vi "xiLIB - PRM_Info.vi"() -> ()   [LabVIEW 2018]
uses:
  Typedefs/xiLIB - PRM_Type.ctl
  Typedefs/xiLIB - PRM_Function.ctl
  xiCam/PRM/PRM/PRM_v2.ctl
panel:
  in  "PRM[]_v2":T1[](array[typedef])=[enum."DEVICE_NAME", enum."DEVICE_TYPE", enum."DEVICE_SN", enum."EXPOSURE", enum."EXPOSURE_MAX", enum."EXPOSURE_MIN", enum."GAIN", enum."GAIN_MAX", enum."GAIN_MIN", enum."DOWNSAMPLING_TYPE", enum."DOWNSAMPLING", enum."DOWNSAMPLING_MAX", enum."DOWNSAMPLING_MIN", enum."IMAGE_DATA_FORMAT", enum."IMAGE_IS_COLOR", enum."COLOR_FILTER_ARRAY", enum."FRAMERATE", enum."FRAMERATE_MAX", enum."FRAMERATE_MIN", enum."BUFFER_POLICY", enum."OFFSET_X", enum."OFFSET_X_MAX", enum."OFFSET_X_MIN", enum."OFFSET_Y", enum."OFFSET_Y_MAX", enum."OFFSET_Y_MIN", enum."WIDTH", enum."WIDTH_MAX", enum."WIDTH_MIN", enum."HEIGHT", enum."HEIGHT_MAX", enum."HEIGHT_MIN", enum."LUT_EN", enum."LUT_INDEX", enum."LUT_INDEX_MAX", enum."LUT_INDEX_MIN", enum."LUT_VALUE", enum."LUT_VALUE_MAX", enum."LUT_VALUE_MIN", enum."TRG_SOURCE", enum."TRG_SOFTWARE", enum."GPI_SELECTOR", enum."GPI_SELECTOR_MAX", enum."GPI_SELECTOR_MIN", enum."GPI_LEVEL", enum."GPI_MODE", enum."GPO_SELECTOR", enum."GPO_SELECTOR_MAX", enum."GPO_SELECTOR_MIN", enum."GPO_MODE", enum."LED_SELECTOR", enum."LED_SELECTOR_MAX", enum."LED_SELECTOR_MIN", enum."LED_MODE", enum."ACQ_BUFFER_SIZE", enum."BUFFERS_QUEUE_SIZE", enum."WB_KR", enum."WB_KG", enum."WB_KB", enum."MANUAL_WB", enum."AUTO_WB", enum."GAMMAY", enum."GAMMAC", enum."SHARPNESS", enum."CC_MATRIX_00", enum."CC_MATRIX_01", enum."CC_MATRIX_02", enum."CC_MATRIX_03", enum."CC_MATRIX_10", enum."CC_MATRIX_11", enum."CC_MATRIX_12", enum."CC_MATRIX_13", enum."CC_MATRIX_20", enum."CC_MATRIX_21", enum."CC_MATRIX_22", enum."CC_MATRIX_23", enum."CC_MATRIX_30", enum."CC_MATRIX_31", enum."CC_MATRIX_32", enum."CC_MATRIX_33", enum."CC_MATRIX_33", enum."AEAG", enum."EXP_PRIORITY", enum."AE_MAX_LIMIT", enum."AG_MAX_LIMIT", enum."AEAG_LEVEL", enum."BPC", enum."DEBOUNCE_EN", enum."DEBOUNCE_T0", enum."DEBOUNCE_T1", enum."DEBOUNCE_POL", enum."IS_COOLED", enum."COOLING", enum."TARGET_TEMP", enum."CHIP_TEMP", enum."LED_SELECTOR_MIN", enum."HDR", enum."LIMIT_BANDWIDTH_MAX", enum."API_VERSION", enum."LUT_EN", enum."AVAILABLE_BANDWIDTH", enum."LIMIT_BANDWIDTH", enum."ACQ_BUFFER_SIZE_UNIT", enum."ACQ_TRANSPORT_BUFFER_COMMIT", enum."AEAG_ROI_HEIGHT", enum."AEAG_ROI_OFFSET_X", enum."AEAG_ROU_OFFSET_Y", enum."AEAG_ROI_WIDTH", enum."SHUTTER_TYPE", enum."GAIN_SELECTOR", enum."SENSOR_FEATURE_SELECTOR", enum."SENSOR_FEATURE_VALUE", enum."OUTPUT_DATA_BIT_DEPTH", enum."IMAGE_DATA_BIT_DEPTH", enum."SENSOR_DATA_BIT_DEPTH", enum."SENSOR_CLOCK_FREQ_HZ", enum."SENSOR_CLOCK_FREQ_INDEX", enum."OUTPUT_DATA_PACKING", enum."OUTPUT_DATA_PACKING_TYPE", enum."TRANSPORT_PIXEL_FORMAT", enum."IMAGE_PAYLOAD_SIZE", enum."SENSOR_TAPS", enum."COLUMN_FPN_CORRECTION", enum."BINNING_HORIZONTAL", enum."BINNING_SELECTOR", enum."BINNING_SELECTOR", enum."BINNING_VERTICAL", enum."DECIMATION_HORIZONTAL", enum."DECIMATION_VERTICAL", enum."DECIMATION_SELECTOR", enum."DECIMATION_VERTICAL"]
  in  "ERROR_CODE[]":i32[](array[numeric])=[0, 1, 2, 3, 4, 5, 6, 7, 8, 9, 10, 11, 12, 13, 14, 15, 16, 17, 18, 19, 20, 21, 22, 23, 24, 25, 26, 27, 28, 29, 30, 31, 32, 33, 34, 35, 36, 38, 39, 40, 41, 42, 43, 44, 45, 46, 47, 48, 49, 50, 51, 52, 53, 54, 55, 100, 101, 103, 104, 105, 106, 107, 108, 109, 110, 111]
  in  "ERROR_DESC[]":string[](array[string])=["Function call succeeded", "Invalid handle", "Register read error", "Register write error", "Freeing resiurces error", "Freeing channel error", "Freeing bandwith error", "Read block error", "Write block error", "No image", "Timeout", "Invalid arguments supplied", "Not supported", "Attach buffers error", "Overlapped result", "Memory allocation error", "DLL context is NULL", "DLL context is non zero", "DLL context exists", "Too many devices connected", "Camera context error", "Unknown hardware", "Invalid TM file", "Invalid TM tag", "Incomplete TM", "Bus reset error", "Not implemented", "Shading too bright", "Shading too dark", "Gain is too low", "Invalid bad pixel list", "Bad pixel list realloc error", "Invalid pixel list", "Invalid Flash File System", "Invalid profile", "Invalid calibration", "Invalid buffer", "Invalid data", "Timing generator is busy", "Wrong operation open/write/read/close", "Acquisition already started", "Old version of device driver installed to the system.", "To get error code please call GetLastError function.", "Data can't be processed", "Acquisition has been stopped. It should be started before GetImage.", "Acquisition has been stoped with error.", "Input ICC profile missed or corrupted", "Output ICC profile missed or corrupted", "Device not ready to operate", "Shading too contrast", "Modile already initialized", "Application doesn't enough privileges(one or more app", "Installed driver not compatible with current software", "TM file was not loaded successfully from resources", "Device has been reseted, abnormal initial state", "Unknown parameter", "Wrong parameter value", "Wrong parameter type", "Wrong parameter size", "Input buffer too small", "Parameter info not supported", "Parameter info not supported", "Data format not supported", "Read only parameter", "No devices found", "This camera does not support currently available bandwidth"]
  in  "PRM-Method[]":T2[](array[typedef])=[enum."Get", enum."Get", enum."Get", enum."Get / Set", enum."Get", enum."Get", enum."Get / Set", enum."Get", enum."Get", enum."Get / Set", enum."Get / Set", enum."Get", enum."Get", enum."Get / Set", enum."Get", enum."Get", enum."Get", enum."Get", enum."Get", enum."Get / Set", enum."Get / Set", enum."Get", enum."Get", enum."Get / Set", enum."Get", enum."Get", enum."Get / Set", enum."Get", enum."Get", enum."Get / Set", enum."Get", enum."Get", enum."Get / Set", enum."Get / Set", enum."Get", enum."Get", enum."Get / Set", enum."Get", enum."Get", enum."Get / Set", enum."Set", enum."Get / Set", enum."Get", enum."Get", enum."Get", enum."Get / Set", enum."Get / Set", enum."Get", enum."Get", enum."Get / Set", enum."Get / Set", enum."Get", enum."Get", enum."Get / Set", enum."Get / Set", enum."Get / Set", enum."Get / Set", enum."Get / Set", enum."Get / Set", enum."Set", enum."Get / Set", enum."Get / Set", enum."Get / Set", enum."Get / Set", enum."Get / Set", enum."Get / Set", enum."Get / Set", enum."Get / Set", enum."Get / Set", enum."Get / Set", enum."Get / Set", enum."Get / Set", enum."Get / Set", enum."Get / Set", enum."Get / Set", enum."Get / Set", enum."Get / Set", enum."Get / Set", enum."Get / Set", enum."Get / Set", enum."Set", enum."Get / Set", enum."Get / Set", enum."Get / Set", enum."Get / Set", enum."Get / Set", enum."Get / Set", enum."Get / Set", enum."Get / Set", enum."Get / Set", enum."Get / Set", enum."Get", enum."Get", enum."Get", enum."Get", enum."Get", enum."Get / Set", enum."Get / Set", enum."Get", enum."Get", enum."Get", enum."Get", enum."Get / Set", enum."Get / Set", enum."Get / Set", enum."Get / Set", enum."Get / Set", enum."Get / Set", enum."Get / Set", enum."Get / Set", enum."Get / Set", enum."Get / Set", enum."Get / Set", enum."Get / Set", enum."Get / Set", enum."Get / Set", enum."Get / Set", enum."Get / Set", enum."Get / Set", enum."Get / Set", enum."Get", enum."Get / Set", enum."Get / Set", enum."Get / Set", enum."Get / Set", enum."Get / Set", enum."Get / Set", enum."Get / Set", enum."Get / Set", enum."Get / Set", enum."Get / Set"]
  in  "PRM-Desc[]":string[](array[string])=["Get camera model name.", "Returns device type (1394, USB2.0, CURRERA…..).", "Returns device serial number in decimal format.", "Set/Get exposure time in microseconds.", "Get longest possible exposure to be set on camera.", "Get shortest possible exposure to be set on camera.", "Set/Get camera gain in dB.", "Get highest possible camera gain in dB.", "Get lowest possible camera gain in dB.", "BINNING: Pixels are interpoled - better image, SKIPPING: pixels are skipped - higher framerate", "Changes image resolution, where one image pixel is: '1' - sensor pixel , '2' - 2x2 , '4' - 4x4.", "Get highest value for binning or skipping.", "Get lowest value for binning or skipping", "Set/Get output image data format. Use class IMG_FORMAT to set value.", "Returns 1 for color cameras", "Returns color filter array type of RAW data.", "Get frames per second.", "Get highest possible framerate for current camera settings.", "Get lowest framerate for current camera settings", "Data move policy", "Set/Get horizontal offset from the origin to the area of interest (in pixels).", "Get maximum horizontal offset from the origin to the area of interest (in pixels).", "Get minimum horizontal offset from the origin to the area of interest (in pixels).", "Set/Get vertical offset from the origin to the area of interest (in pixels).", "Get maximum vertical offset from the origin to the area of interest (in pixels).", "Get minimal vertical offset from the origin to the area of interest (in pixels). ", "Set/Get width of the image provided by the camera (in pixels)", "Get maximal image width provided by the camera (in pixels).", "Get minimal image width provided by the camera (in pixels)", "Set/Get height of the image provided by the camera (in pixels).", "Get maximal image height provided by the camera (in pixels).", "Get minimal image height provided by the camera (in pixels). ", "Activates look up table. Currently available only for Currera-R cameras.", "Controls the index (offset) of the coefficient to access in the LUT.", "Get highest LUT index (offset) of the coefficient to access in the LUT. ", "Get lowest LUT index (offset) of the coefficient to access in the LUT.", "Set/Get value at entry LUTIndex of the LUT.", "Get highest value to be set in LUT.", "Get lowest value to be set in LUT.", "Set/Get source of trigger. Use TRG_SOURCE class to set parameter.", "Set an internal software trigger. PRM.TRG_SOURCE must be set to TRG_SOFTWARE", "Select camera GPI port.", "Get highest GPI port number on camera.", "Get lowest GPI port number on camera.", "Get current GPI level", "Set/Get GPI functionality. Select port by using GPI_SELECTOR parameter. ", "Select camera GPO port", "Get highest GPO port number on camera.", "Get lowest GPI port number on camera", "Set/Get GPO functionality. Select port by using GPO_SELECTOR parameter.", "Selects camera LED to be used. Currently supported only for Currera-R cameras.", "Get highest LED number on camera", "Get lowest LED number on camera", "Set/Get LED functionality. Select port by using LED_SELECTOR parameter", "Acquisition buffer size in bytes.", "Queue of field/frame buffers", "White balance red coefficient. By default 1.", "White balance green coefficient. By default 1.", "White balance blue coefficient. By default 1", "Calculates White Balance. By default -.", "Automatic white balance. By default 0.", "Luminosity gamma. By default 1.0.", "Chromaticity gamma. By default 0.", "Sharpness strenght. By default 0. ", "Color Correction Matrix element [0][0]. By default 1.0", "Color Correction Matrix element [0][1]. By default 0.0", "Color Correction Matrix element [0][2]. By default 0.0", "Color Correction Matrix element [0][3]. By default 0.0.", "Color Correction Matrix element [1][0]. By default 0.0.", "Color Correction Matrix element [1][1]. By default 1.0.", "Color Correction Matrix element [1][2]. By default 0.0.", "Color Correction Matrix element [1][3]. By default 0.0", "Color Correction Matrix element [2][0]. By default 0.0", "Color Correction Matrix element [2][1]. By default 0.0", "Color Correction Matrix element [2][2]. By default 1.0.", "Color Correction Matrix element [2][3]. By default 0.0.", "Color Correction Matrix element [3][0]. By default 0.0", "Color Correction Matrix element [3][1]. By default 0.0. ", "Color Correction Matrix element [3][2]. By default 1.0.", "Color Correction Matrix element [3][3]. By default 0.0", "Set default Color Correction Matrix", "Start automatic exposure/gain. By default 0(disabled).", "Exposure priority (0.5 - exposure 50%, gain 50%). By default 0.8.", "Maximum limit of exposure in AEAG procedure. By default 1000000(1s). ", "Maximum limit of gain in AEAG procedure. By default defined by sensor", "Average intensity of output signal AEAG should achieve(in ). By default 40(). ", "Enable correction of bad pixels. By default 0(disabled).", "Enable/Disable debounce to selected GPI. By default 0(disabled). ", "Debounce time (x * 10us).", "Debounce time (x * 10us).", "Debounce polarity (pol = 1 t0 - falling edge, t1 - rising edge). By default 0(disabled). ", "Returns 1 for cameras that support cooling. By default -", "Set camera cooling. By default 0.", "Set sensor target temperature for cooling. By default 20.", "Camera chip temperature. By default -", "Camera housing tepmerature. By default -.", "Enable High Dynamic Range feature. By default 0(disabled). ", "High Dynamic Range ratio (long exposure time / short exposure time, total exposure time = short + long). By default 4. Type integer", "Return version of xiApi.NET. By default -", "Return version of current device driver. By default -.", "Calculate and return available interface bandwidth(int Megabits).", "Set/get camera data-rate (in Megabits) used for sending image data while acquisition.", "Acquisition buffer size unit in bytes. By default 1. ", "Acquisition transport buffer size in bytes. By default 1048576", "Automatic exposure/gain ROI height. Default depends on sensors resolution and downsampling.", "Automatic exposure/gain ROI offset X. Default 0", "Automatic exposure/gain ROI offset Y. Default 0", "Automatic exposure/gain ROI width. Default Default depends on sensors resolution and downsampling", "Change sensor shutter type(CMOS sensor). Use class SHUTTER_TYPE to set value", "Select gain type to control with GAIN", "Selects the current feature which is accessible by SENSOR_FEATURE_VALUE. Use SENSOR_FEATURE_SELECTOR class to set parameter", "Allows access to sensor feature value currently selected by SENSOR_FEATURE_SELECTOR. All ranges depends on selected feature", "Set/Get device output data bit depth", "Set/Get bitdepth of data returned by function xiGetImage", "Set/Get sensor output data bit depth", "Set/Get sensor clock frequency in Hz.", "Sensor clock frequency. Selects frequency index for sensor. ", "Set/Get Device output data packing (or grouping) enabled. Packing could be enabled if output_data_bit_depth > 8 and packing is available.", "Device output data packing (or grouping) enabled.", "Transport pixel format is format of data transported by link to transport layer.", "Buffer size in bytes sufficient for output image returned by GetImage. Type int. Read only", "Set/Get number of sensor taps. Supported only by MD camera family. ", "Enable correction of column fpn. By default 1(enabled).", "Defines number of horizontal photo-sensitive cells to combine. ", "Defines binning pattern. Use class BINNIG_PATTERN to set value.", "Select Binning engine to configure. Use class BINNIG_SELECTOR to set value.", "Defines number of vertical photo-sensitive cells to combine", "Reduces the horizontal resolution of the image by the specified decimation factor.", "Defines decimation pattern. Use class DECIMATION_PATTERN to set value.", "Select Decimation engine to configure. Use class DECIMATION_SELECTOR to set value.", "Reduces the vertical resolution of the image by the specified decimation factor."]
  in  "PRM-Type[]":T3[](array[typedef])=[enum."String", enum."String", enum."String", enum."Int32", enum."Int32", enum."Int32", enum."Float", enum."Float", enum."Float", enum."DOWNSAMPLING_TYPE", enum."Int32", enum."Int32", enum."Int32", enum."IMAGE_DATA_FORMAT", enum."Int32", enum."Int32", enum."Float", enum."Float", enum."Float", enum."BUFFER_POLICY", enum."Int32", enum."Int32", enum."Int32", enum."Int32", enum."Int32", enum."Int32", enum."Int32", enum."Int32", enum."Int32", enum."Int32", enum."Int32", enum."Int32", enum."Int32", enum."Int32", enum."Int32", enum."Int32", enum."Int32", enum."Int32", enum."Int32", enum."TRG_SOURCE", enum."Int32", enum."Int32", enum."Int32", enum."Int32", enum."Int32", enum."GPI", enum."Int32", enum."Int32", enum."Int32", enum."GPO", enum."Int32", enum."Int32", enum."Int32", enum."LED_MODE", enum."Int32", enum."Int32", enum."Float", enum."Float", enum."Float", enum."Int32", enum."Int32", enum."Float", enum."Float", enum."Float", enum."Float", enum."Float", enum."Float", enum."Float", enum."Float", enum."Float", enum."Float", enum."Float", enum."Float", enum."Float", enum."Float", enum."Float", enum."Float", enum."Float", enum."Float", enum."Float", enum."Int32", enum."Int32", enum."Float", enum."Float", enum."Float", enum."Float", enum."Int32", enum."Int32", enum."Int32", enum."Int32", enum."Int32", enum."Int32", enum."Int32", enum."Float", enum."Float", enum."Float", enum."Float", enum."Int32", enum."String", enum."String", enum."Int32", enum."Int32", enum."Int32", enum."Int32", enum."Int32", enum."Int32", enum."Int32", enum."Int32", enum."SHUTTER_TYPE", enum."GAIN_SELECTOR_TYPE", enum."SENSOR_FEATURE_SELECTOR", enum."Int32", enum."Int32", enum."Int32", enum."Int32", enum."Int32", enum."Int32", enum."Int32", enum."OUTPUT_DATA_PACKING_TYPE", enum."Int32", enum."Int32", enum."Int32", enum."Int32", enum."Int32", enum."BINNING_PATTERN", enum."BINNING_SELECTOR", enum."Int32", enum."Int32", enum."DECIMATION_PATTERN", enum."DECIMATION_SELECTOR", enum."Int32"]
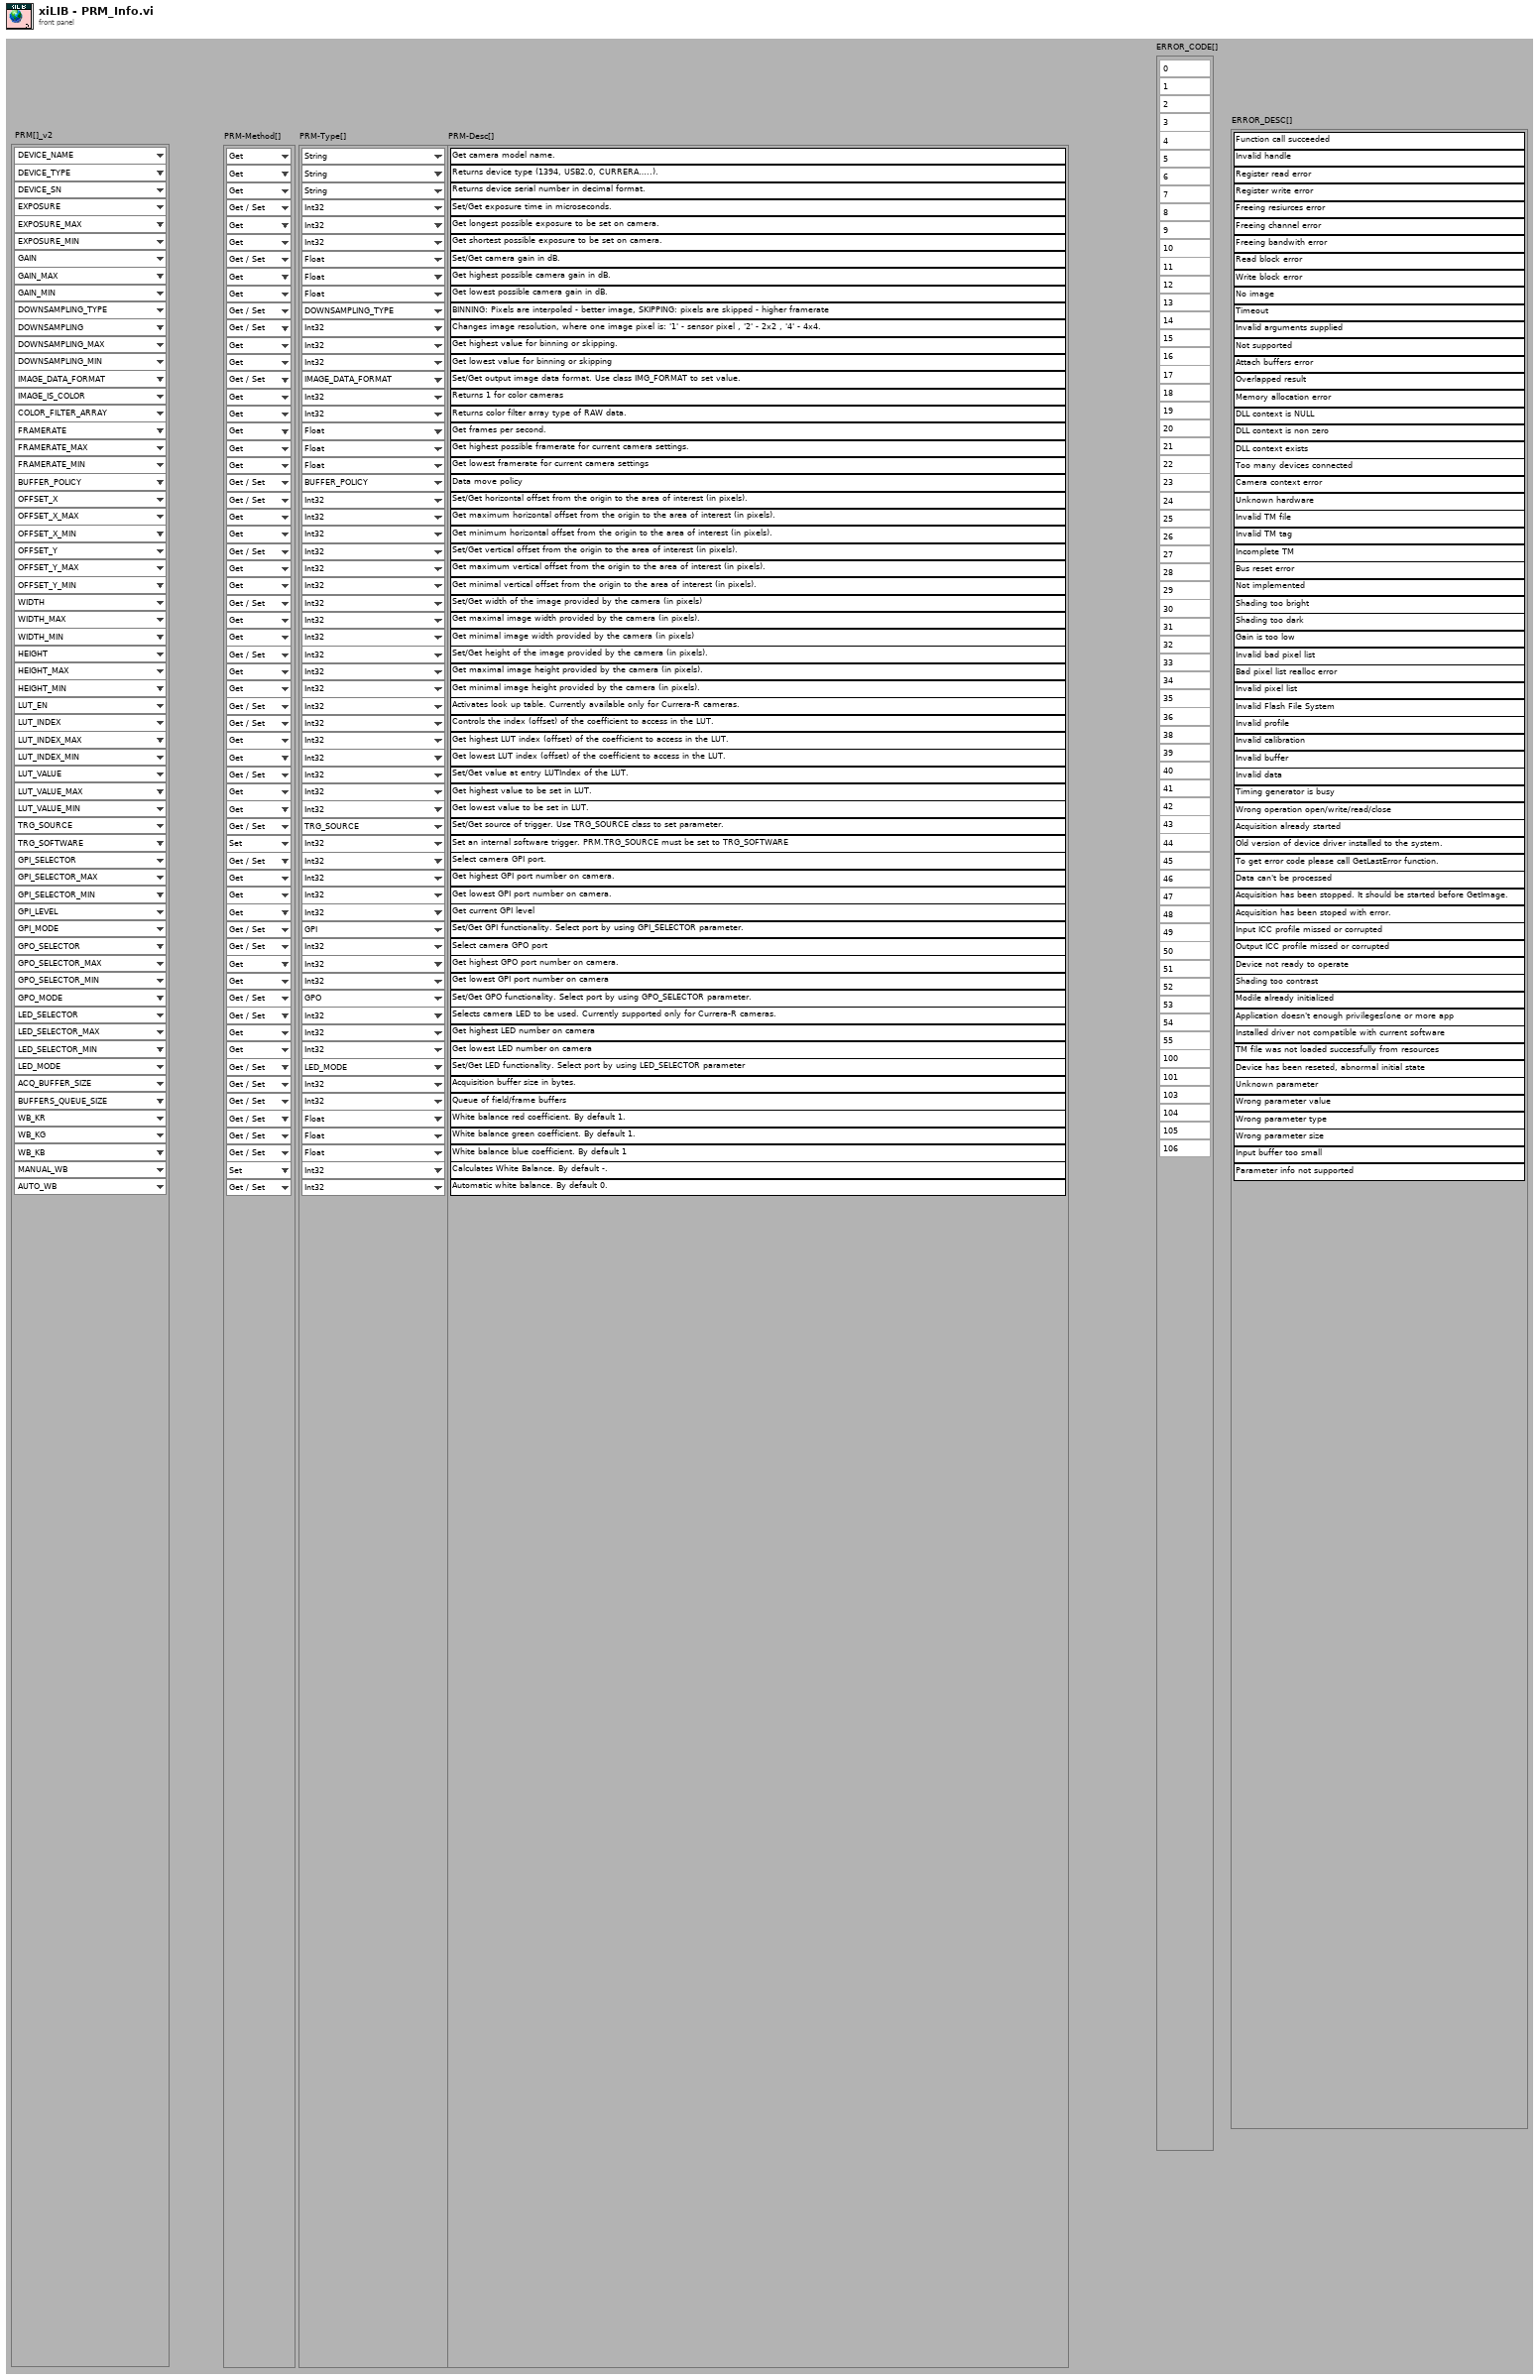
[diagram p1: front panel]
types:
  T1 = typedef "PRM_v2.ctl" = enum16{"ACQ_BUFFER_SIZE", "ACQ_FRAME_BURST_COUNT", "ACQ_TIMING_MODE", "ACQ_TRANSPORT_BUFFER_SIZE", "AE_MAX_LIMIT", "AEAG", "AEAG_LEVEL", "API_VERSION", "AG_MAX_LIMIT", "APPLY_CMS", "AUTO_BANDWIDTH_CALCULATION", "AUTO_WB", "AVAILABLE_BANDWIDTH", "AVAILABLE_BANDWIDTH_MAX", "AVAILABLE_BANDWIDTH_MIN", "BPC", "BUFFER_POLICY", "BUFFERS_QUEUE_SIZE", "CC_MATRIX_00", "CC_MATRIX_01", "CC_MATRIX_02", "CC_MATRIX_03", "CC_MATRIX_10", "CC_MATRIX_11", "CC_MATRIX_12", "CC_MATRIX_13", "CC_MATRIX_20", "CC_MATRIX_21", "CC_MATRIX_22", "CC_MATRIX_23", "CC_MATRIX_30", "CC_MATRIX_31", "CC_MATRIX_32", "CC_MATRIX_33", "CHIP_TEMP", "CMS", "COLOR_FILTER_ARRAY", "COOLING", "DEBOUNCE_EN", "DEBOUNCE_POL", "DEBOUNCE_T0", "DEBOUNCE_T1", "DEBUG_LEVEL", "DEFAULT_CC_MATRIX", "DEVICE_INSTANCE_PATH", "DEVICE_MODEL_ID", "DEVICE_NAME", "DEVICE_SN", "DEVICE_TYPE", "DEVICE_USER_ID", "DOWNSAMPLING", "DOWNSAMPLING_MAX", "DOWNSAMPLING_MIN", "DOWNSAMPLING_TYPE", "DRV_VERSION", "EXP_PRIORITY", "EXPOSURE", "EXPOSURE_DIRECT_UPDATE", "EXPOSURE_MAX", "EXPOSURE_MIN", "FFS_FILE_NAME", "FPGA1_VERSION", "FRAMERATE", "FRAMERATE_MAX", "FRAMERATE_MIN", "FREE_FFS_SIZE", "GAIN", "GAIN_DIRECT_UPDATE", "GAIN_MAX", "GAIN_MIN", "GAMMAC", "GAMMAY", "GPI_LEVEL", "GPI_MODE", "GPI_SELECTOR", "GPI_SELECTOR_MAX", "GPI_SELECTOR_MIN", "GPO_MODE", "GPO_SELECTOR", "GPO_SELECTOR_MAX", "GPO_SELECTOR_MIN", "HDR", "HDR_T1", "HDR_T2", "HEIGHT", "HEIGHT_MAX", "HEIGHT_MIN", "HOUSE_TEMP", "IMAGE_DATA_FORMAT", "IMAGE_IS_COLOR", "INPUT_CMS_PROFILE", "IS_COOLED", "IS_DEVICE_EXIST", "KNEEPOINT1", "KNEEPOINT2", "LED_MODE", "LED_SELECTOR", "LED_SELECTOR_MAX", "LED_SELECTOR_MIN", "LIMIT_BANDWIDTH", "LIMIT_BANDWIDTH_MAX", "LIMIT_BANDWIDTH_MIN", "LUT_EN", "LUT_INDEX", "LUT_INDEX_MAX", "LUT_INDEX_MIN", "LUT_VALUE", "LUT_VALUE_MAX", "LUT_VALUE_MIN", "MANUAL_WB", "MCU1_VERSION", "MCU2_VERSION", "OFFSET_X", "OFFSET_X_MAX", "OFFSET_X_MIN", "OFFSET_Y", "OFFSET_Y_MAX", "OFFSET_Y_MIN", "OUTPUT_CMS_PROFILE", "OUTPUT_DATA_BIT_DEPTH", "OUTPUT_DATA_PACKING", "READ_FILE_FFS", "RECENT_FRAME", "SENSOR_DATA_BIT_DEPTH", "SENSOR_MODE", "SENSOR_TAPS", "SHARPNESS", "SHUTTER_TYPE", "TARGET_TEMP", "TRG_DELAY", "TRG_SELECTOR", "TRG_SOFTWARE", "TRG_SOURCE", "USED_FFS_SIZE", "WB_KB", "WB_KG", "WB_KR", "WIDTH", "WIDTH_MAX", "WIDTH_MIN", "WRITE_FILE_FFS", "ACQ_BUFFER_SIZE_UNIT", "ACQ_TRANSPORT_BUFFER_COMMIT", "AEAG_ROI_HEIGHT", "AEAG_ROI_OFFSET_X", "AEAG_ROU_OFFSET_Y", "AEAG_ROI_WIDTH", "API_CONTEXT_LIST", "BINNING_HORIZONTAL", "BINNING_SELECTOR", "BINNING_VERTICAL", "COLUMN_FPN_CORRECTION", "COUNTER_SELECTOR", "COUNTER_VALUE", "DECIMATION_HORIZONTAL", "DECIMATION_SELECTOR", "DECIMATION_VERTICAL", "DEVICE_ID", "DEVICE_LOCATION_PATH", "DEVICE_MANIFEST", "DEVICE_RESET", "DEVICE_SENS_SN", "EXPOSURE_BURST_COUNT", "FFS_ACCESS_KEY", "GAIN_SELECTOR", "HW_REVISION", "IMAGE_BLACK_LEVEL", "IMAGE_DATA_BIT_DEPTH", "IMAGE_DATA_FORMAT_RGB32_ALPHA", "IMAGE_PAYLOAD_SIZE", "LENS_APERTURE_VALUE", "LENS_FEATURE", "LENS_FEATURE_SELECTOR", "LENS_FOCAL_LENGTH", "LENS_FOCUS_DISTANCE", "LENS_FOCUS_MOVE", "LENS_FOCUS_MOVEMENT_VALUE", "LENS_MODE", "OUTPUT_DATA_PACKING_TYPE", "SENSOR_CLOCK_FREQ_HZ", "SENSOR_CLOCK_FREQ_INDEX", "SENSOR_FEATURE_SELECTOR", "SENSOR_FEATURE_VALUE", "SENSOR_OUTPUT_CHANNEL_COUNT", "TRANSPORT_PIXEL_FORMAT", "TS_RST_MODE", "TS_RST_SOURCE"}
  T2 = typedef "xiLIB - PRM_Function.ctl" = enum16{"Get / Set", "Get", "Set"}
  T3 = typedef "xiLIB - PRM_Type.ctl" = enum16{"Int32", "Float", "String", "DOWNSAMPLING_TYPE", "IMAGE_DATA_FORMAT", "BUFFER_POLICY", "TRG_SOURCE", "GPI", "GPO", "ACQ_TIMING_MODE", "BINNING_PATTERN", "BINNING_SELECTOR", "CMS_MODE", "COUNTER_SELECTOR", "DEBUG_LEVEL", "DECIMATION_PATTERN", "DECIMATION_SELECTOR", "GAIN_SELECTOR_TYPE", "LED_MODE", "LENS_FEATURE_SELECTOR", "LENS_MODE", "OUTPUT_DATA_PACKING_TYPE", "SENSOR_FEATURE_SELECTOR", "SHUTTER_TYPE", "TRG_SELECTOR", "TS_RST_MODE", "TS_RST_SOURCE"}
diagram:
